vi "Cam-color2.vi"(7 "error in":errorcluster) -> (20 "Classifier Session (Color Classification 1)":T2, 21 "Classes (Color Classification 1)":string[](array[string]), 27 "error out":errorcluster)   [LabVIEW 2018]
uses:
  <vilib>/vision/Classification.llb/IMAQ Classifier Session.ctl
  <vilib>/vision/Classification.llb/IMAQ Classifier Read Options.ctl
  <vilib>/vision/NI_Vision_Development_Module.lvlib
panel:
  out "Image Out":T1(plugin-control)
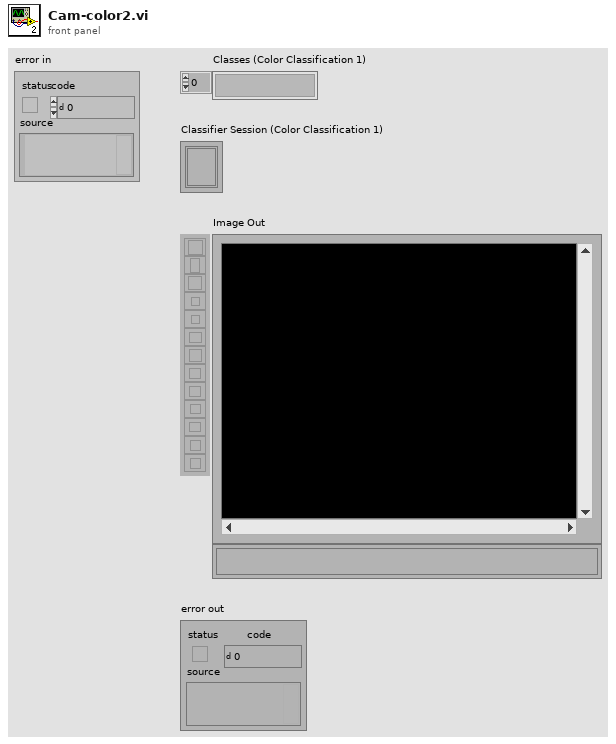
[diagram p1: front panel]
types:
  T1 = typedef "IMAQ Image.ctl" = refnum<image>
  T2 = typedef "IMAQ Classifier Session.ctl" = refnum<k1>
  T3 = cluster{"Global Rectangle":i32[], "Contours":cluster{"ID":enum32{"External", "Internal"}, "Type":u32, "Coordinates":i32[]}[]}
  T4 = typedef "IMAQ Classifier Read Options.ctl" = i32
  T5 = typedef "ROI Descriptor" = cluster{"Global Rectangle":i32[], "Contours":cluster{"ID":enum32{"External", "Internal"}, "Type":u32, "Coordinates":i32[]}[]}
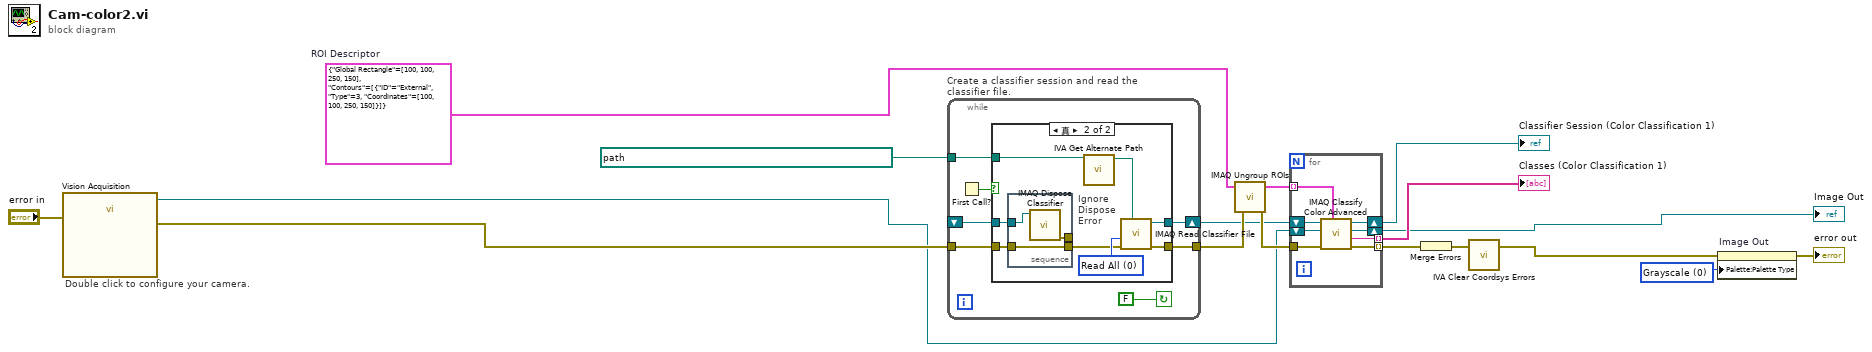
[diagram p0: block diagram]
diagram:
  w1 = u32 0 items=["Grayscale", "Binary", "Gradient", "Rainbow", "Temperature", "User Defined", "Binary 16 Bit", "Gradient 16 Bit", "Rainbow 16 Bit", "Temperature 16 Bit", "User Defined 16 Bit"] ("Palette Type")
  w13 = T3 {"Global Rectangle"=[100, 100, 250, 150], "Contours"=[{"ID"=enum."External", "Type"=3, "Coordinates"=[100, 100, 250, 150]}]}  # ROI Descriptor
  # "Double click to configure your camera."
  n1 = call "Vision Acquisition"("error in"="error in") -> ("Image Out"=w6:T1, "error out"=w16:errorcluster)  [unwired: 25 in]
  n2 = while "Create a classifier session and read the classifier file." {
    shift-right: [w24] -> w5
    shift-left: _ -> [w23]
    tunnel: w16 -> [w21]
    tunnel: [w20] -> w12
    tunnel: path "D:/Labviewprogram/视觉/视觉框架/Color 识别.clf" ("File Path") -> [w19]
    stop <- FALSE continue-if-true
    n3 = First Call?() -> (First Call?: T/F=w18:bool)
    n4 = case "条件结构" shown="真" w18 {
      tunnel: [w26 w33] -> w24
      tunnel: w23 -> [w26 w31]
      tunnel: w21 -> [w25 w30]
      tunnel: [w25 w32] -> w20
      tunnel: w19 -> [_ w28]
      frame False {
      }
      frame True {
        w34 = T4 0 items=["Read All", "Add Samples, Do Not Change Options", "Read Options, Do Not Add Samples"] ("Read Options")
        # "Ignore Dispose Error"
        n5 = stacked-sequence "层叠式顺序结构" {
          tunnel: w31 -> [w37]
          tunnel: w30 -> [w36]
          tunnel: [w36] -> w29
          tunnel: [w35] -> _
          frame #0 {
            n6 = call "IMAQ Dispose Classifier"("Classifier Session"=w37) -> ("error out"=w35:errorcluster)  [unwired: 1 in, 9 out]
          }
        }
        n7 = call <vilib>:"IVA Get Alternate Path.vi"("Path In"=w28) -> ("Path Out"=w27:path)  [unwired: 10 out]
        n8 = call "IMAQ Read Classifier File"("File Path"=w27, "error in (no error)"=w29, "Read Options"=w34) -> ("error out"=w32:errorcluster, "Classifier Session"=w33:T2)  [unwired: 1 in, 6 out]
      }
    }
  }
  n9 = call "IMAQ Ungroup ROIs"("error in (no error)"=w12, "ROI Descriptor"=w13) -> ("error out"=w11:errorcluster, "ROI Descriptors out"=w10:T5[])  [unwired: 2 out]
  n10 = for "For循环" {
    tunnel: [w45] -> w14 mode=indexing
    tunnel: [w44] -> w9 mode=indexing
    tunnel: w11 -> [w42]
    tunnel: w10 -> [w41] mode=indexing
    shift-right: [w39] -> w2
    shift-left: w6 -> [w40]
    shift-right: [w38] -> w4
    shift-left: w5 -> [w43]
    n11 = call "IMAQ Classify Color Advanced"("ROI Descriptor"=w41, "error in (no error)"=w42, "Image"=w40, "Classifier Session"=w43) -> ("error out"=w44:errorcluster, "Class"=w45:string, "Image (dup)"=w39:T1, "Classifier Session (dup)"=w38:T2)  [unwired: 4 out]
  }
  "Classes (Color Classification 1)" <- w14
  "Classifier Session (Color Classification 1)" <- w4
  "Image Out" <- w2
  n12 = Merge Errors(w9) -> (w8:errorcluster)
  n13 = call <vilib>:"IVA Clear Coordsys Errors.vi"("error in (no error)"=w8) -> ("error out"=w7:errorcluster)  [unwired: 10 in]
  n14 = property on="Image Out" class="ImageControl"(error in=w7, "Palette:Palette Type"=w1) -> (error out=→"error out":errorcluster)  [unwired: 1 in, 1 out]
